vi "Store Value as Variable.vi"(9 "Value":dbl, 10 "Position":u32, 11 "Variable Name":string) -> ()   [LabVIEW 2015, in "Measurement.lvclass"]
uses:
  Measurement.lvclass
  <vilib>/Cree, Inc/Cree Test Framework/Core Launcher/Core Manager Methods -- Enum.ctl
  <vilib>/Cree, Inc/Cree Test Framework/Core Launcher/Core Launcher.lvlib
  <vilib>/Cree, Inc/Cree Test Framework/Classes/Variable Engine/Class/Variable Engine.lvclass
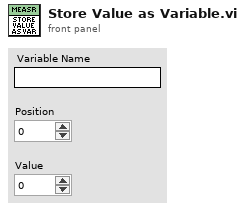
[diagram p1: front panel]
types:
  T1 = typedef "Core Launcher.lvlib/Core Manager Methods -- Enum.ctl" = enum16{"Spawn Objects", "Get Objects", "Destroy Objects"}
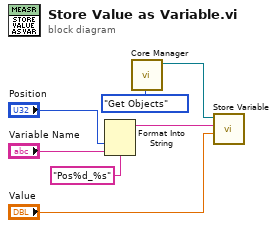
[diagram p0: block diagram]
diagram:
  n1 = Format Into String(format string="Pos%d_%s", "Position", "Variable Name") -> (resulting string=w4:string)  [unwired: 2 in, 1 out]
  n2 = call <vilib>:"Core Manager.vi"("Method"=Core_Manager_Methods_--_Enum."Get Objects") -> ("Variable Engine"=w2:refnum<class "Variable Engine.lvclass">)  [unwired: 6 in, 4 out]
  n3 = call <vilib>:"Store Variable.vi"("Value"="Value", "Key"=w4, "Acrobat Template in"=w2) -> ()  [unwired: 7 in, 2 out]
